vi "Write Element of Sounds.vi"(9 "Sound.lvclass":refnum<class "Sound.lvclass">=refnum, 10 "index":i32, 11 "Aggregate Sound in":refnum<class "Aggregate Sound.lvclass">=refnum) -> (3 "Aggregate Sound out":refnum<class "Aggregate Sound.lvclass">)   [LabVIEW 2010, in "Aggregate Sound.lvclass"]
uses:
  Aggregate Sound.lvclass
  Sound/Sound.lvclass
  Aggregate Sound.lvclass/Aggregate Sound.ctl
  Silence/Silence.lvclass
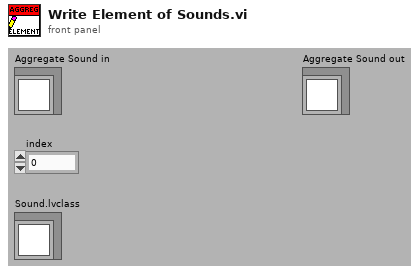
[diagram p1: front panel]
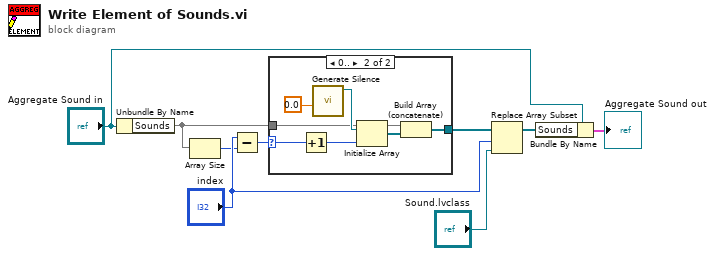
[diagram p0: block diagram]
diagram:
  n1 = Unbundle By Name("Aggregate Sound in") -> ("Sounds"=w5)
  n2 = Array Size(array=w5) -> (size(s)=w3:i32)
  n3 = Subtract(x="index", y=w3) -> (x-y=w2:i32)
  n4 = case shown="0.." w2 {
    selector: w2 -> [_ w15]
    tunnel: w5 -> [w10 w14]
    tunnel: [w10 w12] -> w1
    frame Default {
    }
    frame 0.. {
      n5 = Increment(x=w15) -> (x+1=w11:i32)
      n6 = call "Generate Silence.vi"("Duration (1 second)"=0.0) -> ("Silence out"=w16:refnum<class "Silence.lvclass">)  [unwired: 10 in]
      n7 = Initialize Array(w16, w11) -> (w13:refnum<class "Silence.lvclass">[])
      n8 = Build Array (concatenate)(w14, w13) -> (w12:refnum<class "Silence.lvclass">[])
    }
  }
  n9 = Replace Array Subset(array=w1, new element="Sound.lvclass", index="index") -> (w6:refnum<class "Sound.lvclass">[])
  n10 = Bundle By Name(cluster="Aggregate Sound in", "Sounds"=w6) -> (→"Aggregate Sound out":cluster{})
